vi "TimeDateInfo.vi"(0 "refnum":refnum<file>, 11 "offset":i32) -> (2 "Time/Date Info":cluster{"date":string, "time":string}, 4 "dup refnum":refnum<file>, 6 "date":string, 8 "time":string)   [LabVIEW 2022 SP3]
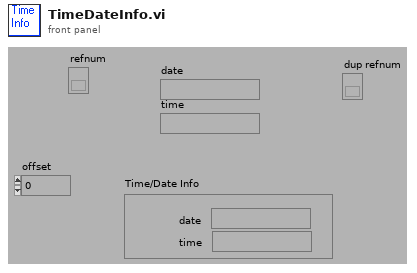
[diagram p1: front panel]
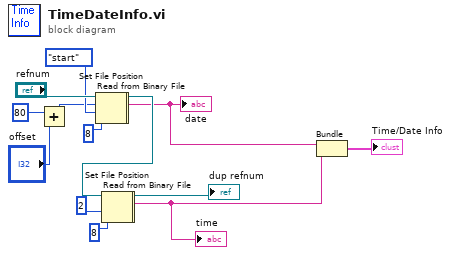
[diagram p0: block diagram]
diagram:
  n1 = Add(x=80 ("pos offset (0)"), y="offset") -> (x+y=w6:i32)
  n2 = Set File Position(offset (in bytes) (0)=w6, refnum="refnum", from (0:start)=enum16{"start", "end", "current"}."start" ("pos mode (0:2)")) -> (refnum out=w2:refnum<file>, error out=w1:errorcluster)  [unwired: 1 in]
  n3 = Read from Binary File(8:w1, 10:8 ("count"), 11:w2) -> (2:w10:string, 3:w12:refnum<file>)  [unwired: 5 out]
  "date" <- w10
  n4 = Set File Position(refnum=w12, from (0:start)=2) -> (refnum out=w4:refnum<file>, error out=w3:errorcluster)  [unwired: 1 in, 1 out]
  n5 = Read from Binary File(8:w3, 10:8 ("count"), 11:w4) -> (2:w9:string, 3:→"dup refnum":refnum<file>)  [unwired: 5 out]
  "time" <- w9
  n6 = Bundle(w10, w9) -> (→"Time/Date Info":cluster{string, string})  [unwired: 1 out]
